vi "enumerate.vi"(8 "Path In":path=path "C:/Users/loa/Desktop/data", 11 "Name Time Date In":string="im_spec_") -> (0 "Path Out":path=path "C:/Users/loa/Desktop/data", 3 "Complete File Name Out":string, 4 "path error out":errorcluster)   [LabVIEW 2014]
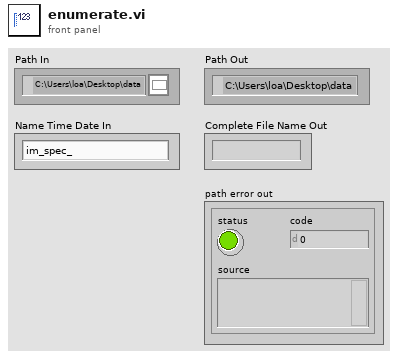
[diagram p1: front panel]
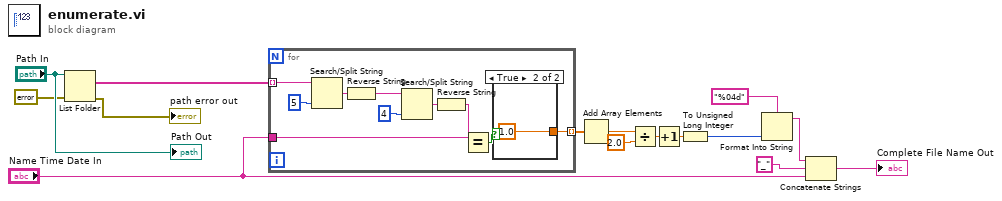
[diagram p0: block diagram]
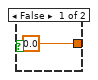
[diagram p2: hidden frame]
diagram:
  n1 = List Folder(path="Path In", error in=errorcluster {"status"=FALSE, "code"=0, "source"=""}) -> (filenames=w3:string[], error out=→"path error out":errorcluster)  [unwired: 2 in, 2 out]
  n2 = for {
    tunnel: w3 -> [w17] mode=indexing
    tunnel: [w25] -> w4 mode=indexing
    tunnel: "Name Time Date In" -> [w24]
    n3 = Search/Split String(string=w17, offset (0)=5) -> (match + rest of string=w20:string)  [unwired: 1 in, 2 out]
    n4 = Reverse String(1:w20) -> (0:w19:string)
    n5 = Search/Split String(string=w19, offset (0)=4) -> (match + rest of string=w18:string)  [unwired: 1 in, 2 out]
    n6 = Reverse String(1:w18) -> (0:w16:string)
    n7 = Equal?(x=w24, y=w16) -> (x = y?=w23:bool)
    n8 = case shown="True" w23 {
      tunnel: [0.0 1.0 ("x")] -> w25
      frame False {
      }
      frame True {
      }
    }
  }
  n9 = Add Array Elements(numeric array=w4) -> (sum=w10:dbl)
  n10 = Divide(x=w10, y=2.0) -> (x/y=w9:dbl)
  n11 = Increment(x=w9) -> (x+1=w15:dbl)
  n12 = To Unsigned Long Integer(number=w15) -> (unsigned 32bit integer=w8:u32)
  n13 = Format Into String(format string="%04d", w8) -> (resulting string=w6:string)  [unwired: 2 in, 1 out]
  n14 = Concatenate Strings(w6, "_" ("string"), "Name Time Date In") -> (→"Complete File Name Out":string)
  "Path Out" <- "Path In"
